vi "User Dynamic (multiple).vi"(7 "User.Example.lvclass":refnum<class "User.Example.lvclass">, 8 "error in (no error)":errorcluster, 11 "XY-data":cluster{"X-array":dbl[], "Y-array":dbl[]}[](array[cluster]) {"Y-array" format="%.2p"; "X-array" format="%.2p"}) -> (0 "error out":errorcluster, 3 "XY-data out":cluster{"X-array":dbl[], "Y-array":dbl[]}[](array[cluster]) {"Y-array" format="%.2p"; "X-array" format="%.2p"}, 5 "User.Example.lvclass out":refnum<class "User.Example.lvclass">)   [LabVIEW 2019, in "User.Example.lvclass"]
uses:
  User.Example.lvclass
  User/User.lvclass
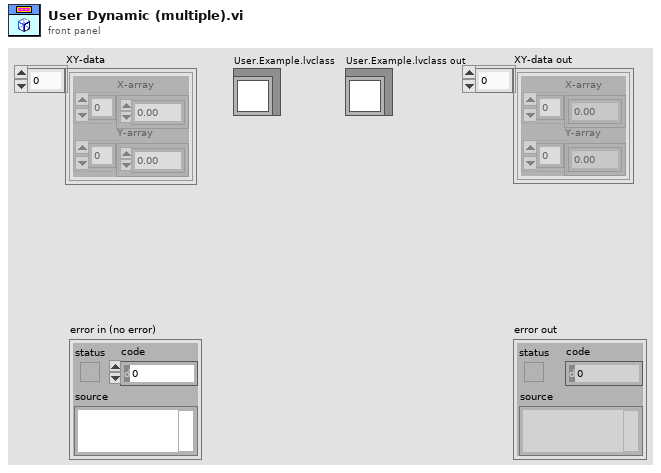
[diagram p1: front panel]
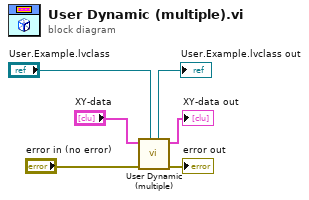
[diagram p0: block diagram]
diagram:
  n1 = call-parent "User Dynamic (multiple).vi"("User.lvclass"="User.Example.lvclass", "error in (no error)"="error in (no error)", "XY-data"="XY-data") -> ("error out"=→"error out":errorcluster, "XY-data out"=→"XY-data out":cluster{"X-array":dbl[], "Y-array":dbl[]}[], "User.lvclass out"=→"User.Example.lvclass out":refnum<class "User.Example.lvclass">)  [unwired: 6 in]
